vi "Get Autorange Spanfactors and Offsets.vi"(8 "error in (no error)":errorcluster caption="Fehler (Eingang, kein Fehler)", 9 "Autorange Bereiche":T1[](array[typedef]), 10 "Offset":sgl[](array[numeric]), 11 "Span":sgl[](array[numeric])) -> (0 "error out":errorcluster caption="Fehler (Ausgang)", 2 "Autorange Offsets":string[](array[string]), 3 "Autorange Spanfactors":string[](array[string]), 4 "Autorange Offsets":string, 5 "Autorange Spanfactors":string)   [LabVIEW 2020, in "Linearisierung v2.lvlib"]
uses:
  Linearisierung v2.lvlib
  Visualisierungs Elemente/Auswahlfeld.ctl
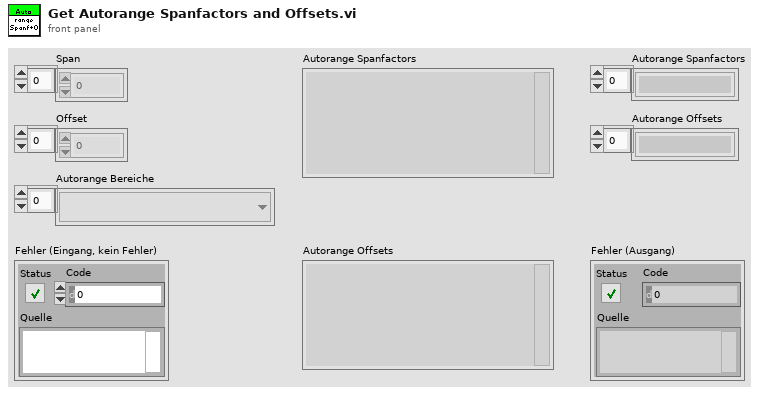
[diagram p1: front panel]
types:
  T1 = typedef "Auswahlfeld.ctl" = u16
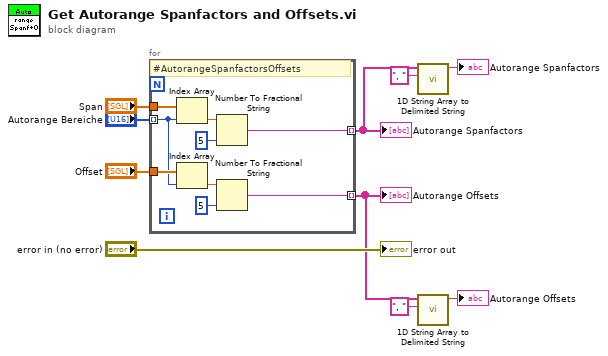
[diagram p0: block diagram]
diagram:
  n1 = for {
    tunnel: "Span" -> [w17]
    tunnel: "Autorange Bereiche" -> [w12] mode=indexing
    tunnel: [w16] -> w6 mode=indexing
    tunnel: "Offset" -> [w13]
    tunnel: [w11] -> w1 mode=indexing
    # "#AutorangeSpanfactorsOffsets"
    n2 = Index Array(array=w17, index=w12) -> (element=w19:sgl)
    n3 = Index Array(array=w13, index=w12) -> (element=w14:sgl)
    n4 = Number To Fractional String(number=w19, precision (6)=i16 5 ("Genauigkeit (6)")) -> (F-format string=w16:string)  [unwired: 2 in]
    n5 = Number To Fractional String(number=w14, precision (6)=i16 5 ("Genauigkeit (6)")) -> (F-format string=w11:string)  [unwired: 2 in]
  }
  "Autorange Offsets" <- w1
  "Autorange Spanfactors" <- w6
  n6 = call <vilib>:"1D String Array to Delimited String.vi"("delimiter"=", ", "string array"=w6) -> ("delimited string"=→"Autorange Spanfactors":string)  [unwired: 9 in]
  n7 = call <vilib>:"1D String Array to Delimited String.vi"("delimiter"=", ", "string array"=w1) -> ("delimited string"=→"Autorange Offsets":string)  [unwired: 9 in]
  "error out" <- "error in (no error)"
